vi "micro_2.vi"(6 "result":string, 7 "Type":string, 8 "err":bool, 9 "SN":string, 10 "version":string, 11 "PN":string) -> (3 "Chaîne":string)   [LabVIEW 2020]
panel:
  out "error out":errorcluster
  in  "errin":errorcluster
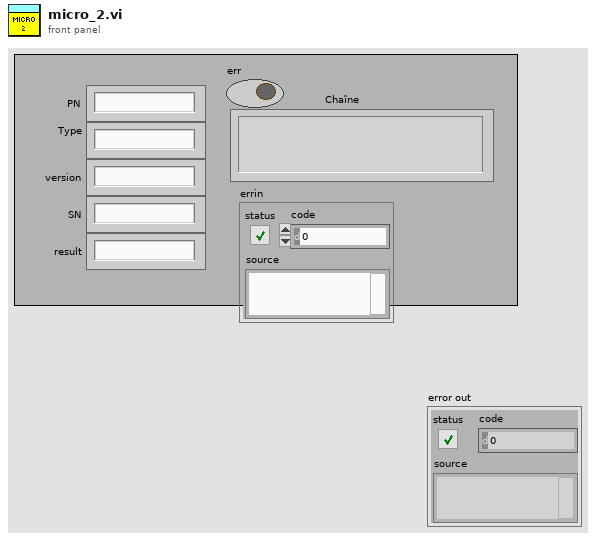
[diagram p1: front panel]
types:
  T1 = enum16{"open", "replace", "create", "open or create", "replace or create", "replace or create with confirmation"}
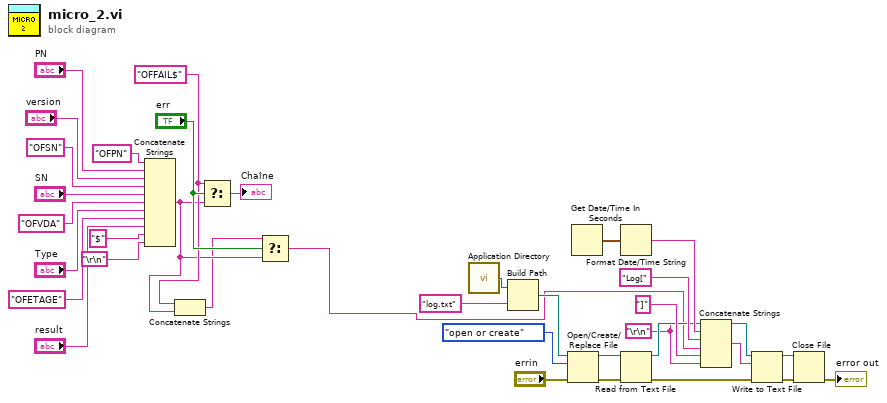
[diagram p0: block diagram]
diagram:
  w6 = "\r\n"
  w3 = "OFFAIL$" ("t")
  n1 = Concatenate Strings("OFPN" ("chaîne"), "PN", "version", "OFSN" ("chaîne"), "SN", "OFVDA" ("chaîne"), "Type", "OFETAGE" ("chaîne"), "result", "$" ("chaîne"), "\r\n") -> (w2:string)
  n2 = Concatenate Strings(w3, w2) -> (w1:string)
  n3 = Select(t=w3, s="err", f=w2) -> (s? t:f=→"Chaîne":string)
  n4 = Select(t=w1, s="err", f=w2) -> (s? t:f=w4:string)
  n5 = call <vilib>:"Application Directory.vi"() -> ("Application Directory"=w22:path)
  n6 = Build Path ("Composer un chemin")(base path=w22, name or relative path="log.txt") -> (appended path=w21:path)
  n7 = Open/Create/Replace File(file path (use dialog)=w21, error in="errin", operation (0:open)=T1."open or create") -> (refnum out=w9:refnum<file>, error out=w10:errorcluster)  [unwired: 3 in, 1 out]
  n8 = Get Date/Time In Seconds() -> (seconds since 1Jan1904=w15:timestamp)
  n9 = Format Date/Time String(seconds (now)=w15) -> (date/time string=w14:string)  [unwired: 2 in]
  n10 = Read from Text File(file (use dialog)=w9, error in=w10) -> (refnum out=w8:refnum<file>, error out=w11:errorcluster)  [unwired: 2 in, 2 out]
  n11 = Concatenate Strings(w6, w14, "Log[" ("string"), w4, "]" ("string"), w6) -> (w7:string)
  n12 = Write to Text File(file (use dialog)=w8, text=w7, error in=w11) -> (refnum out=w16:refnum<file>, error out=w18:errorcluster)  [unwired: 1 in, 1 out]
  n13 = Close File(refnum=w16, error in=w18) -> (error out=→"error out":errorcluster)  [unwired: 1 out]
